vi "DecoderGetBall.vi"(8 "error in":errorcluster, 9 "Array":u8[](array[numeric]) format="%02x") -> (0 "error out":errorcluster, 1 "array w/ subset deleted":u8[](array[numeric]), 3 "ball":T1)   [LabVIEW 2017]
uses:
  Core/AI Ball.ctl
panel:
  in  "element":T1
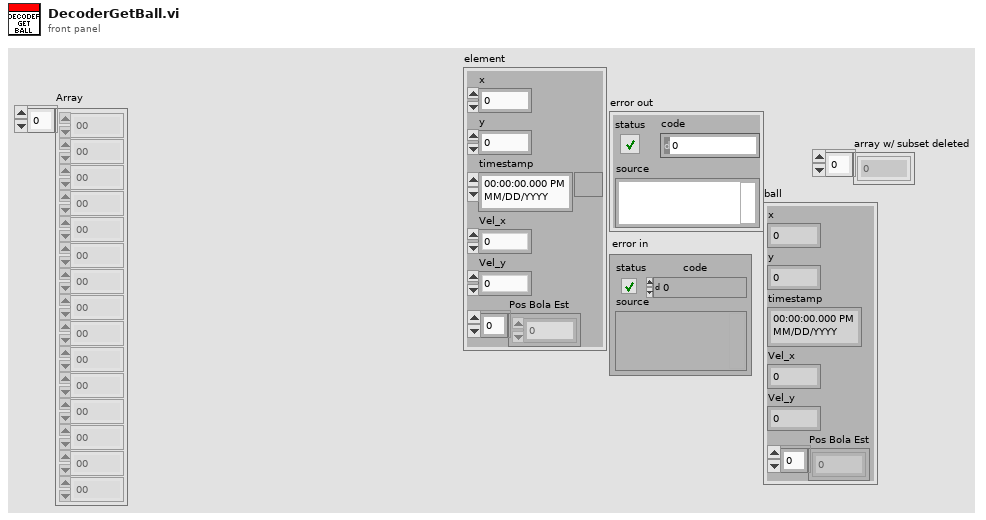
[diagram p1: front panel]
types:
  T1 = typedef "AI Ball.ctl" = cluster{"x":dbl, "y":dbl, "timestamp":timestamp, "Vel_x":dbl, "Vel_y":dbl, "Pos Bola Est":dbl[]}
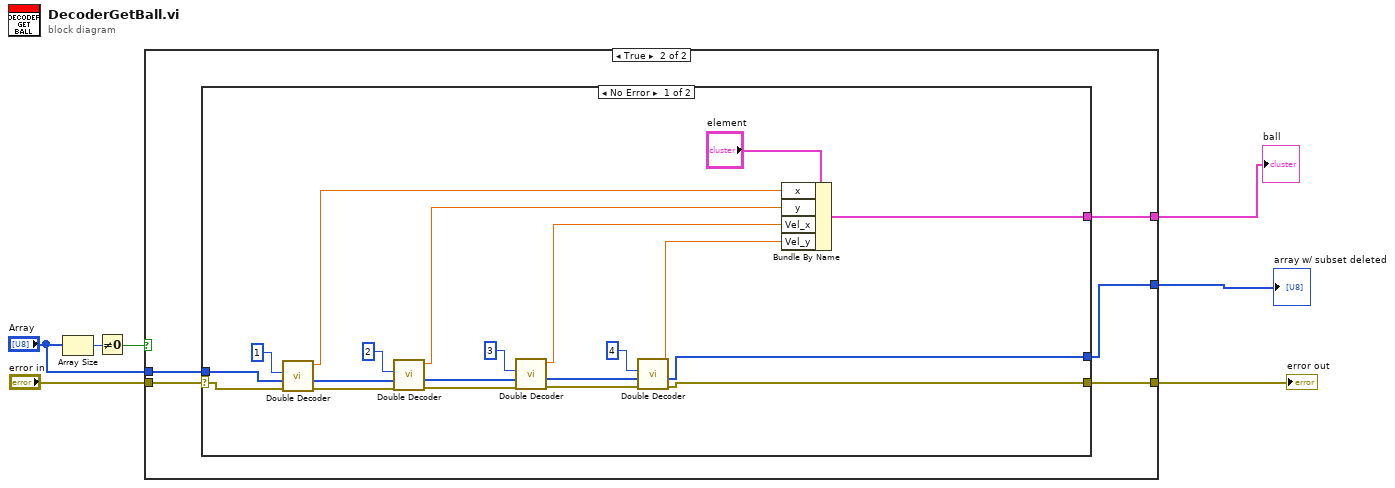
[diagram p0: block diagram]
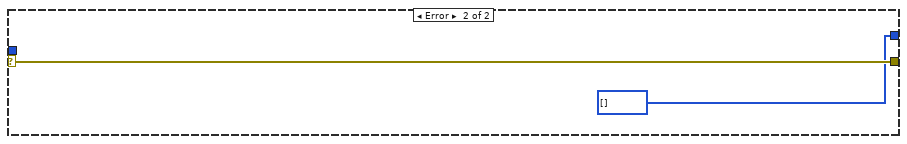
[diagram p3: hidden frame]
diagram:
  n1 = Array Size(array="Array") -> (size(s)=w5:i32)
  n2 = Not Equal To 0?(x=w5) -> (x != 0?=w3:bool)
  n3 = case shown="True" w3 {
    tunnel: "error in" -> [_ w12]
    tunnel: "Array" -> [_ w11]
    tunnel: [_ w10] -> w4
    tunnel: [_ w9] -> w2
    tunnel: [_ w8] -> w1
    frame False {
    }
    frame True {
      n4 = case shown="No Error" w12 {
        selector: w12 -> [w31 w34]
        tunnel: [w20 w34] -> w10
        tunnel: [w19 u8[] [] ("array w/ subset deleted")] -> w9
        tunnel: w11 -> [w32 _]
        tunnel: [w13 _] -> w8
        frame No Error {
          n5 = call "Double Decoder.vi"("error in (no error)"=w31, "Array"=w32, "Key"=1) -> ("error out"=w25:errorcluster, "array w/ subset deleted"=w26:u8[], "Double"=w17:dbl)  [unwired: 5 in, 1 out]
          n6 = call "Double Decoder.vi"("error in (no error)"=w25, "Array"=w26, "Key"=2) -> ("error out"=w23:errorcluster, "array w/ subset deleted"=w24:u8[], "Double"=w16:dbl)  [unwired: 5 in, 1 out]
          n7 = call "Double Decoder.vi"("error in (no error)"=w23, "Array"=w24, "Key"=3) -> ("error out"=w21:errorcluster, "array w/ subset deleted"=w22:u8[], "Double"=w15:dbl)  [unwired: 5 in, 1 out]
          n8 = call "Double Decoder.vi"("error in (no error)"=w21, "Array"=w22, "Key"=4) -> ("error out"=w20:errorcluster, "array w/ subset deleted"=w19:u8[], "Double"=w14:dbl)  [unwired: 5 in, 1 out]
          n9 = Bundle By Name(cluster="element", "x"=w17, "y"=w16, "Vel_x"=w15, "Vel_y"=w14) -> (w13:T1)
        }
        frame Error {
        }
      }
    }
  }
  "error out" <- w4
  "array w/ subset deleted" <- w2
  "ball" <- w1
